vi "Calculation_Tracks_Statistics-4.vi"(8 "error IN":errorcluster, 9 "[IN] Tracks Statistics":T1, 10 "[IN] Filtered Tracks":cluster{"Tracks":dbl[], "Start Pos":i32}[](array[cluster]), 11 "[IN] Movie Values":T3 {"Particle Fil Setups"."Type of particle filter"."Measurement Parameter" items=["Center of Mass X", "Center of Mass Y", "First Pixel X", "First Pixel Y", "Bounding Rect Left", "Bounding Rect Top", "Bounding Rect Right", "Bounding Rect Bottom", "Max Feret Diameter Start X", "Max Feret Diameter Start Y", "Max Feret Diameter End X", "Max Feret Diameter End Y", "Max Horiz. Segment Length Left", "Max Horiz. Segment Length Right", "Max Horiz. Segment Length Row", "-", "Bounding Rect Width", "Bounding Rect Height", "Bounding Rect Diagonal", "Perimeter", "Convex Hull Perimeter", "Holes' Perimeter", "Max Feret Diameter", "Equivalent Ellipse Major Axis", "Equivalent Ellipse Minor Axis", "Equivalent Ellipse Minor Axis (Feret)", "Equivalent Rect Long Side", "Equivalent Rect Short Side", "Equivalent Rect Diagonal", "Equivalent Rect Short Side (Feret)", "Average Horiz. Segment Length", "Average Vert. Segment Length", "Hydraulic Radius", "Waddel Disk Diameter", "-", "Area", "Holes' Area", "Particle & Holes' Area", "Convex Hull Area", "Image Area", "-", "Number of Holes", "Number of Horiz. Segments", "Number of Vert. Segments", "-", "Orientation", "Max Feret Diameter Orientation", "-", "% Area/Image Area", "% Area/(Particle & Holes' Area)", "Ratio of Equivalent Ellipse Axes", "Ratio of Equivalent Rect Sides", "-", "Elongation Factor", "Compactness Factor", "Heywood Circularity Factor", "Type Factor", "-", "Sum X", "Sum Y", "Sum XX", "Sum XY", "Sum YY", "Sum XXX", "Sum XXY", "Sum XYY", "Sum YYY", "-", "Moment of Inertia XX", "Moment of Inertia XY", "Moment of Inertia YY", "Moment of Inertia XXX", "Moment of Inertia XXY", "Moment of Inertia XYY", "Moment of Inertia YYY", "Norm. Moment of Inertia XX", "Norm. Moment of Inertia XY", "Norm. Moment of Inertia YY", "Norm. Moment of Inertia XXX", "Norm. Moment of Inertia XXY", "Norm. Moment of Inertia XYY", "Norm. Moment of Inertia YYY", "Hu Moment 1", "Hu Moment 2", "Hu Moment 3", "Hu Moment 4", "Hu Moment 5", "Hu Moment 6", "Hu Moment 7"]}) -> (0 "error OUT":errorcluster, 1 "[OUT] Tracks Statistics":T1)   [LabVIEW 2013]
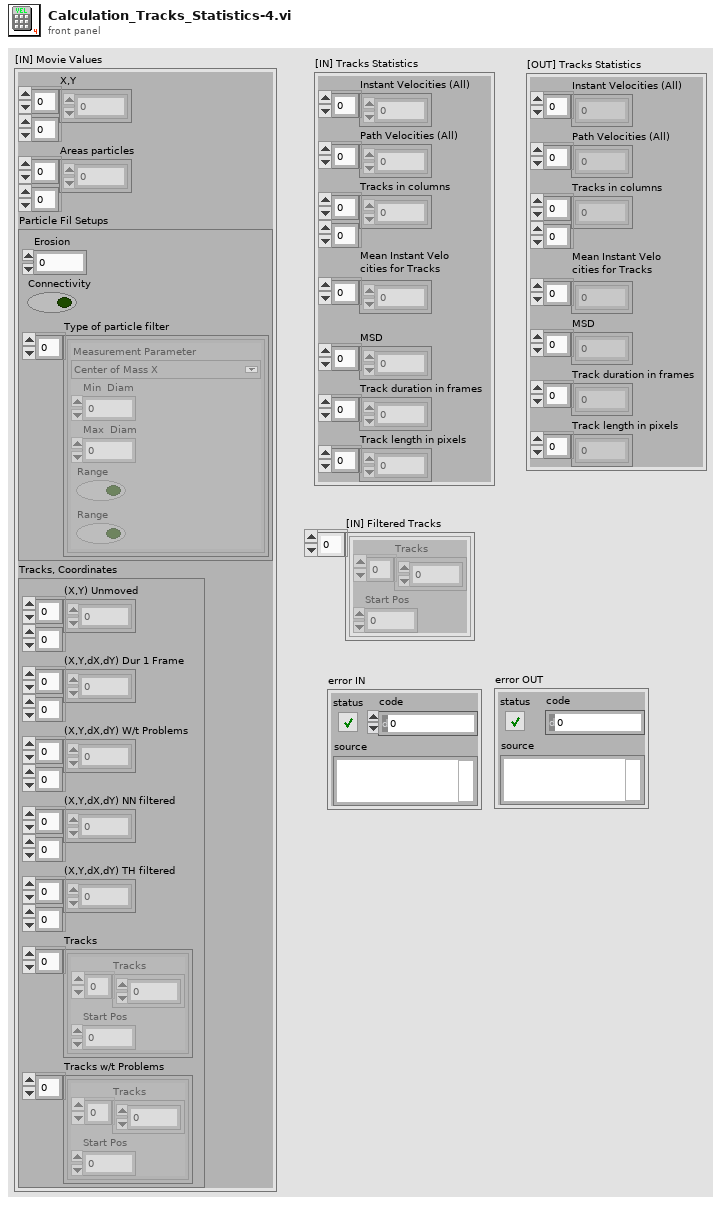
[diagram p1: front panel]
types:
  T1 = cluster{"Instant Velocities (All)":dbl[], "Path Velocities (All) ":dbl[], "Tracks in columns":dbl[][], "Mean Instant Velo\ncities for Tracks":dbl[], "MSD":dbl[], "Track duration in frames":u16[], "Track length in pixels":dbl[]}
  T2 = typedef "Particle Parameters" = i32
  T3 = cluster{"X,Y":dbl[][], "Areas particles":dbl[][], "Particle Fil Setups":cluster{"Erosion":i32, "Connectivity ":bool, "Type of particle filter":cluster{"Measurement Parameter":T2, "Min  Diam":dbl, "Max  Diam":dbl, "Range":bool, "Range":bool}[]}, "Tracks, Coordinates":cluster{"(X,Y) Unmoved":dbl[][], "(X,Y,dX,dY) Dur 1 Frame":dbl[][], "(X,Y,dX,dY) W/t Problems":dbl[][], "(X,Y,dX,dY) NN filtered":dbl[][], "(X,Y,dX,dY) TH filtered":dbl[][], "Tracks":cluster{"Tracks":dbl[], "Start Pos":i32}[], "Tracks w/t Problems":cluster{"Tracks":dbl[], "Start Pos":i32}[]}}
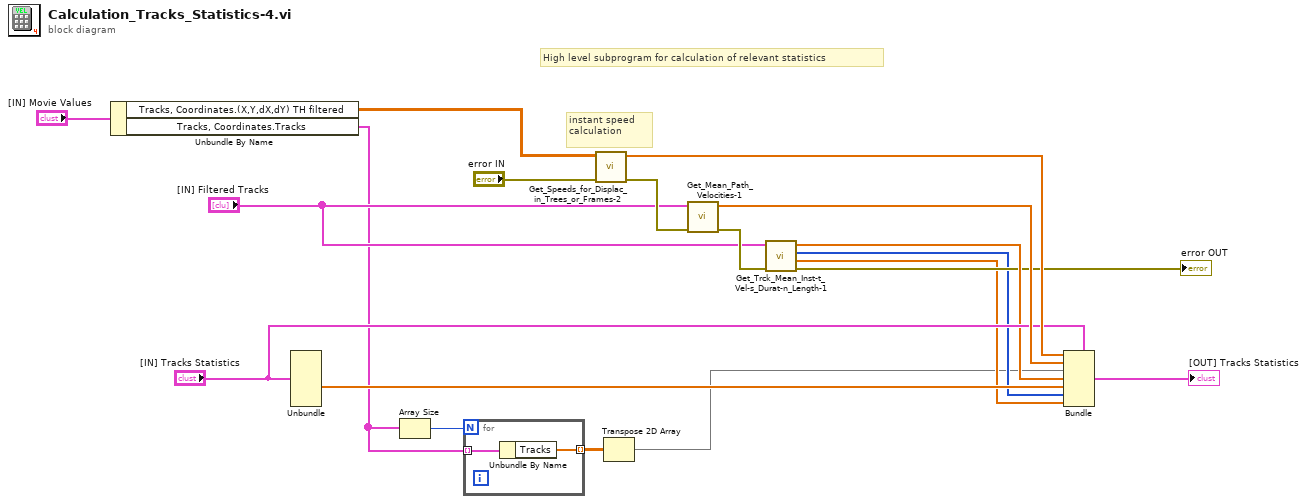
[diagram p0: block diagram]
diagram:
  # "High level subprogram for calculation of relevant statistics"
  # "instant speed \ncalculation"
  n1 = Unbundle By Name("[IN] Movie Values") -> ("Tracks, Coordinates.(X,Y,dX,dY) TH filtered"=w5:dbl[][], "Tracks, Coordinates.Tracks"=w4:cluster{"Tracks":dbl[], "Start Pos":i32}[])
  n2 = Unbundle("[IN] Tracks Statistics") -> ("MSD"=w18:dbl[])  [unwired: 6 out]
  n3 = Array Size(array=w4) -> (size(s)=w1:i32)
  n4 = for {
    N: w1 -> [_]
    tunnel: w4 -> [w21] mode=indexing
    tunnel: [w20] -> w3 mode=indexing
    n5 = Unbundle By Name(w21) -> ("Tracks"=w20:dbl[])
  }
  n6 = call "Get_Speeds_for_Displac_in_Trees_or_Frames-2.vi"("error IN"="error IN", "[IN] Displacements in Frame-to-\nFrame Manner or in Tracks (Trees)"=w5) -> ("error OUT"=w16:errorcluster, "[OUT] Velocities\nin (pixel/frame)"=w17:dbl[])  [unwired: 4 in]
  n7 = Transpose 2D Array(2D array=w3) -> (transposed array=w2:dbl[][])
  n8 = call "Get_Mean_Path_Velocities-1.vi"("error IN"=w16, "[IN] Tracks + Starting Position"="[IN] Filtered Tracks") -> ("error OUT"=w12:errorcluster, "[OUT] Mean Path Velocities"=w15:dbl[])  [unwired: 4 in]
  n9 = call "Get_Trck_Mean_Inst-t_Vel-s_Durat-n_Length-1.vi"("error IN"=w12, "[IN] Tracks + Starting Position"="[IN] Filtered Tracks") -> ("error OUT"=→"error OUT":errorcluster, "[OUT] Track length"=w7:dbl[], "[OUT] Track Duration"=w8:u16[], "[OUT] Mean Instant Vel-s"=w10:dbl[])  [unwired: 2 in]
  n10 = Bundle(cluster="[IN] Tracks Statistics", "Instant Velocities (All)"=w17, "Path Velocities (All)"=w15, "Tracks in columns"=w2, "Mean Instant Velo\ncities for Tracks"=w10, "MSD"=w18, "Track duration in frames"=w8, "Track length in pixels"=w7) -> (→"[OUT] Tracks Statistics":T1)
